vi "Requests.vi"(8 "error in (no error)":errorcluster, 9 "write enable":bool=TRUE, 11 "ICPCON ET-7051 in":refnum<class "ICPCON ET-7051.lvclass">) -> (0 "error out":errorcluster, 3 "ICPCON ET-7051 out":refnum<class "ICPCON ET-7051.lvclass">)   [LabVIEW 2021, in "ICPCON ET-7051.lvclass"]
uses:
  ICPCON ET-7051.lvclass
  D:/my_projects/projects/Algorithms/Labview/21/Master CR/Master CR.lvclass
  D:/my_projects/projects/Algorithms/Labview/21/Master CR/Devices/ET7000/TCP/TCP.lvclass
  Master CR.lvclass/Master CR.ctl
  Modbus_v121c/Modbus Data Unit/Modbus Data Unit.lvclass/Modbus Data Unit.ctl
  Modbus_v121c/Network Protocol/Network Master/Network Master.lvclass/Network Master.ctl
  Network Protocol/Read Network Protocol.vi
  Modbus_v121c/Master Function Definition/Read Discrete Inputs Request.vi
  Modbus_v121c/Network Protocol/Network Master/Read write Master.vi
  Modbus_v121c/Master Function Definition/Read Discrete Inputs Response.vi
  Modbus_v121c/Modbus Data Unit/Construct PDU.vi
  Modbus_v121c/Utility/Bytes to Bits.vi
  Modbus_v121c/Master Function Definition/Function code mismatch error.vi
  Modbus_v121c/Data Model/Error Generator.vi
  Modbus_v121c/Modbus Data Unit/Deconstruct PDU.vi
  TCP/TCP.lvclass
  Modbus_v121c/Network Protocol/Network Master/Network Master.lvclass
  Modbus_v121c/Modbus Data Unit/Modbus Data Unit.lvclass
  Modbus_v121c/Data Model/Device Data Model.lvclass
  Modbus_v121c/Transmission Data Unit/Transmission Data Unit.lvclass
  Master CR.lvclass
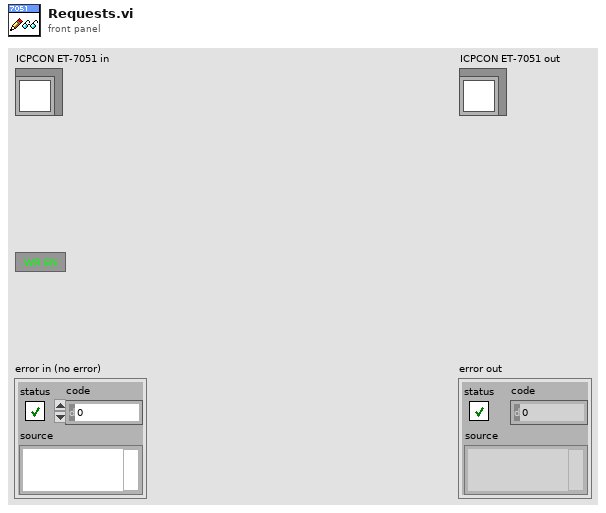
[diagram p1: front panel]
types:
  T1 = typedef "Device Data Model.lvclass/N channel.ctl" = cluster{"N DI channel":i32, "N DO channel":i32, "N AI channel":i32, "N AO channel":i32}
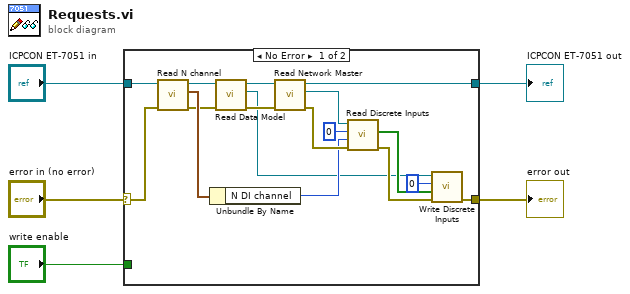
[diagram p0: block diagram]
diagram:
  n1 = case shown="No Error" "error in (no error)" {
    selector: "error in (no error)" -> [w19 w24]
    tunnel: [w10 w24] -> w2
    tunnel: [w16 w23] -> w4
    tunnel: "ICPCON ET-7051 in" -> [w21 w23]
    tunnel: "write enable" -> [_ _]
    frame No Error {
      n2 = call "Read N channel.vi"("error in (no error)"=w19, "Master CR in"=w21) -> ("error out"=w18:errorcluster, "N channel"=w22:T1, "Master CR out"=w20:refnum<class "ICPCON ET-7051.lvclass">)  [unwired: 7 in]
      n3 = Unbundle By Name(w22) -> ("N DI channel"=w11:i32)
      n4 = call "Read Data Model.vi"("error in (no error)"=w18, "Master CR in"=w20) -> ("error out"=w15:errorcluster, "Data Model"=w6:refnum<class "Device Data Model.lvclass">, "Master CR out"=w17:refnum<class "ICPCON ET-7051.lvclass">)  [unwired: 7 in]
      n5 = call "Read Network Master.vi"("error in (no error)"=w15, "TCP in"=w17) -> ("error out"=w13:errorcluster, "Network Master"=w12:refnum<class "Network Master.lvclass">, "TCP out"=w16:refnum<class "ICPCON ET-7051.lvclass">)  [unwired: 7 in]
      n6 = call "Read Discrete Inputs.vi"("error in (no error)"=w13, "number of discrete inputs"=w11, "starting address"=u16 0, "Modbus master in"=w12) -> ("error out"=w9:errorcluster, "discrete input values"=w8:bool[])  [unwired: 5 in, 1 out]
      n7 = call-dynamic "Write Discrete Inputs.vi"("error in (no error)"=w9, "input values"=w8, "starting address"=u16 0, "Device Data Model in"=w6) -> ("error out"=w10:errorcluster)  [unwired: 6 in, 1 out]
    }
    frame Error {
    }
  }
  "error out" <- w2
  "ICPCON ET-7051 out" <- w4
